vi "example (Express VI).vi"() -> ()   [LabVIEW 2021]
uses:
  <vilib>/Analysis/2dsp.llb/Power Spectrum (DBL).vi
  <vilib>/Analysis/NI_AALPro.lvlib
panel:
  in  "Frequency":dbl=10.1
  in  "Delay Time (s)":dbl=1.0
  out "Waveform Graph":dbl[](graph)
  in  "stop":bool
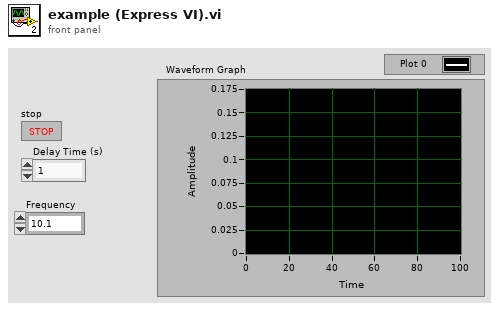
[diagram p1: front panel]
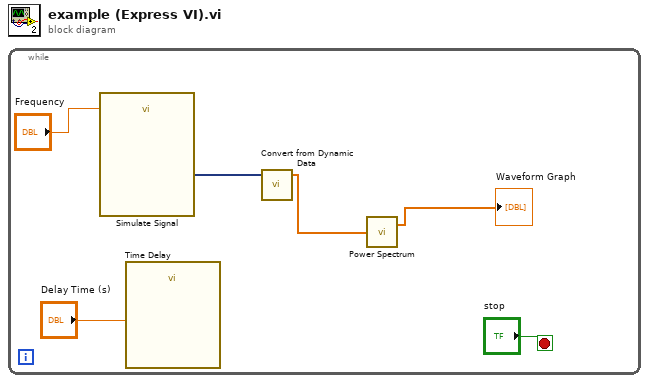
[diagram p0: block diagram]
diagram:
  n1 = while {
    stop <- "stop" stop-if-true
    n2 = call "Simulate Signal"("Frequency"="Frequency") -> ("Triangle"=w6:dynamicdata)  [unwired: 13 in, 1 out]
    n3 = call "Time Delay"("Delay Time (s)"="Delay Time (s)") -> ()  [unwired: 10 in, 1 out]
    n4 = call "Convert from Dynamic Data"("Dynamic Data Type"=w6) -> ("Array"=w3:dbl[])  [unwired: 3 in]
    n5 = call-poly <vilib>:"Power Spectrum.vi"("X"=w3) -> ("Power Spectrum"=→"Waveform Graph":dbl[])  [unwired: 1 out]
  }
